vi "Generate Tamer Status.vi"(8 "error in (no error)":errorcluster, 11 "Monkey in":refnum<class "Tamer.lvclass">) -> (0 "error out":errorcluster, 2 "Tamer Panel":T1, 3 "Monkey out":refnum<class "Tamer.lvclass">)   [LabVIEW 2020, in "TALOS.lvlib" / "Tamer.lvlib" / "Tamer.lvclass"]
uses:
  Tamer.lvclass
  C:/LabVIEW Code/TALOS/talos/Father of all uServices/Father of all uServices/Father of all uServices.lvclass
  Tamer Status.ctl
  Monkey Summary.ctl
  Run Utilities/TypeDefs/Monkey Status.ctl
  Link Chain GUI.ctl
  Tamer.lvclass/Tamer.ctl
  Ancestor/Ancestor/Ancestor.lvclass/Ancestor.ctl
  Support VIs/Generate Error.vi
  FGV/Error Memory/Get Error Description.vi
  Support VIs/Get PC name.vi
  Ancestor/Ancestor/Read ID.vi
  Support VIs/Get Class Name.vi
  <vilib>/Utility/error.llb/Clear Errors.vi
  FGV/Error Memory/Error Memory Core.vi
  <vilib>/AdvancedString/Delimited String to 1D String Array.vi
  Support VIs/Circus Root Path.vi
  FGV/Error Memory/Error Crt Lvl checker.vi
  FGV/Error Memory/Error Memory Core.vi/40c8088d-b597-4017-91af-faa98e00292e.vi
  FGV/Error Memory/Error Memory Core.vi/d4a3ab98-063c-4e44-b43d-fbdcfe6c2be2.vi
  Father of all uServices/Father of all uServices/Children Methods/Get GUI Item Value - Variant.vi
  Support VIs/Global Memory.vi
  <vilib>/Utility/LVClass/Get LV Class Name.vi
  Support VIs/Is in Packed Library.vi
  Support VIs/TALOS Root path.vi
  Support VIs/Read CSV worksheet.vi
  Support VIs/Global Constants.vi
  <vilib>/Utility/error.llb/General Error Handler.vi
  Support VIs/Error Log.vi
  Ancestor/Ancestor/Ancestor.lvclass
  <vilib>/Comparison/Equal/Equal Functor/Equal Functor.lvclass
  Father of all uServices/Father of all uServices/Father of all uServices.lvclass
  TALOS.lvlib
  C:/LabVIEW Code/TALOS/talos/Ancestor/Ancestor/Ancestor.lvclass
  C:/LabVIEW Code/TALOS/builds/Actor Framework PPL/Actor Framework.lvlibp/1abvi3w/vi.lib/ActorFramework/Actor/Actor.lvclass
  C:/LabVIEW Code/TALOS/talos/Internal uServices/System uServices/Tamer/Tamer.lvclass
  Run Utilities/Run Utilities.lvlib
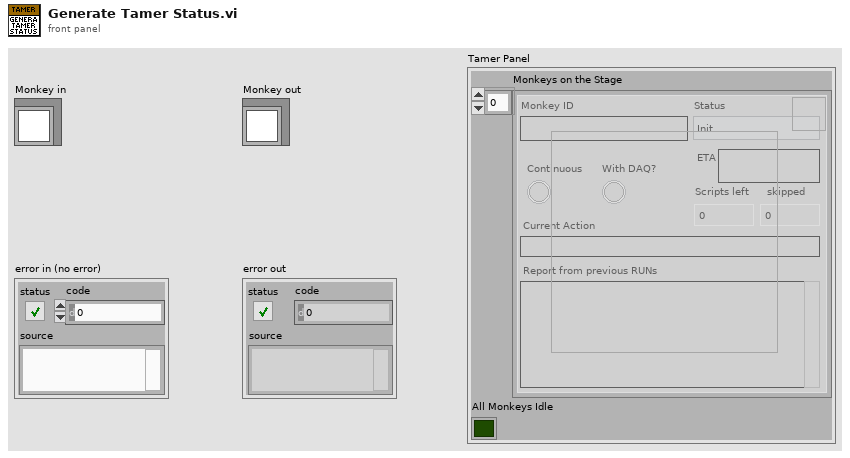
[diagram p1: front panel]
types:
  T1 = typedef "TALOS.lvlib/Tamer.lvlib/Tamer.lvclass/Tamer Status.ctl" = cluster{"Monkeys on the Stage":T2[], "All Monkeys Idle":bool}
  T2 = typedef "TALOS.lvlib/Tamer.lvlib/Tamer.lvclass/Monkey Summary.ctl" = cluster{"Color":u32, "Status":T3, "Continuous":bool, "Scripts left":u32, "Scripts skipped":u32, "ETA":string, "Current Action":string, "Report from previous RUNs":string, "Monkey ID":string, "With DAQ?":bool, "Linked?":T4, "Paused":bool}
  T3 = typedef "TALOS.lvlib/Run Utilities.lvlib/Monkey Status.ctl" = enum16{"Init", "Paused", "Ongoing", "Stopped", "Finished (no errors)", "Finished (with errors)"}
  T4 = typedef "TALOS.lvlib/Tamer.lvlib/Tamer.lvclass/Link Chain GUI.ctl" = bool
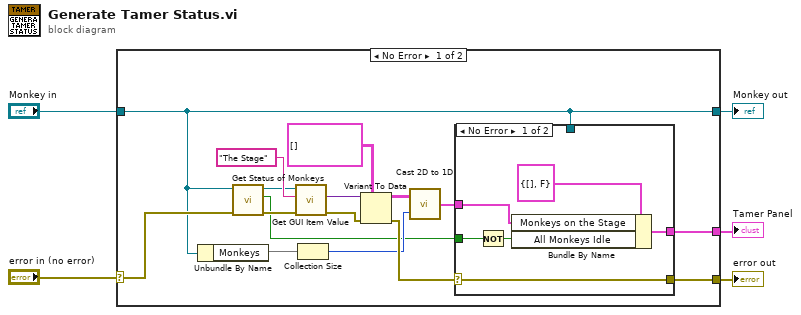
[diagram p0: block diagram]
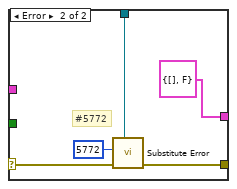
[diagram p2: hidden frame]
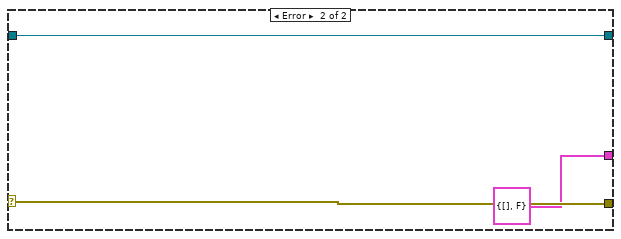
[diagram p3: hidden frame]
diagram:
  n1 = case shown="No Error" "error in (no error)" {
    selector: "error in (no error)" -> [w13 w35]
    tunnel: [w9 w35] -> w4
    tunnel: "Monkey in" -> [w8 w34]
    tunnel: [w8 w34] -> w2
    tunnel: [w10 T1 {"Monkeys on the Stage"=[], "All Monkeys Idle"=FALSE} ("Tamer Panel")] -> w1
    frame No Error {
      n2 = Unbundle By Name(w8) -> ("Monkeys"=w16:map{string, string[]})
      n3 = call-dynamic "Get Status of Monkeys.vi"("error in (no error)"=w13, "Tamer in"=w8) -> ("error out"=w12:errorcluster, "Anything running?"=w11:bool, "Tamer out"=w7:refnum<class "Tamer.lvclass">)  [unwired: 7 in]
      n4 = call-poly "Get GUI Item Value.vi"("error in (no error)"=w12, "FP Item Name"="The Stage", "uService Template in"=w7) -> ("error out"=w20:errorcluster, "Value"=w21:variant)  [unwired: 6 in, 1 out]
      n5 = Collection Size(1:w16) -> (0:w15:i32)
      n6 = Variant To Data(error in=w20, type=T2[][] [] ("The Stage"), Variant=w21) -> (data=w18:T2[][], error out=w17:errorcluster)
      n7 = call "Cast 2D to 1D.vi"("1D size"=w15, "2D Synchronous Monkeys"=w18) -> ("1D Synchronous Monkeys"=w14:T2[])
      n8 = case shown="No Error" w17 {
        selector: w17 -> [w22 w31]
        tunnel: w14 -> [w26 _]
        tunnel: w11 -> [w25 _]
        tunnel: [w23 T1 {"Monkeys on the Stage"=[], "All Monkeys Idle"=FALSE} ("Tamer Panel")] -> w10
        tunnel: [w22 w30] -> w9
        tunnel: w8 -> [_ w29]
        frame No Error {
          n9 = Not(x=w25) -> (.not. x?=w24:bool)
          n10 = Bundle By Name(cluster=T1 {"Monkeys on the Stage"=[], "All Monkeys Idle"=FALSE} ("Tamer Panel"), "Monkeys on the Stage"=w26, "All Monkeys Idle"=w24) -> (w23:T1)
        }
        frame Error {
          # "#5772"
          n11 = call "Substitute Error.vi"("LabVIEW Object"=w29, "error in (no error)"=w31, "Error Code"=5772) -> ("error out"=w30:errorcluster)  [unwired: 8 in]
        }
      }
    }
    frame Error {
    }
  }
  "Monkey out" <- w2
  "error out" <- w4
  "Tamer Panel" <- w1
